vi "Update DelaysHW.vi"(8 "error in (no error)":errorcluster, 11 "BME_DG_System in":refnum<class "BME_DG_System.lvclass">) -> (0 "error out":errorcluster, 3 "BME_DG_System out":refnum<class "BME_DG_System.lvclass">)   [LabVIEW 2009, in "POLARIS BME DG.lvlib" / "BME_DG_System.lvclass"]
uses:
  BME_DG_System.lvclass
  BME_DG_System.lvclass/BME_DG_System.ctl
  BME_DG_Base/BME_DG_Base.lvclass
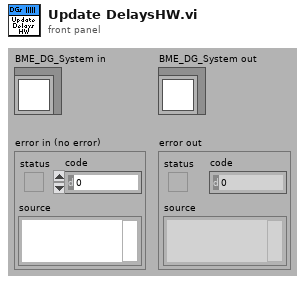
[diagram p1: front panel]
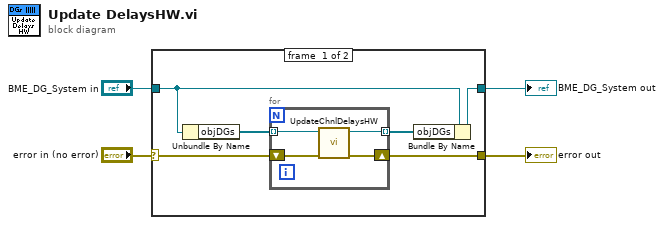
[diagram p0: block diagram]
diagram:
  n1 = case shown="No Error" "error in (no error)" {
    selector: "error in (no error)" -> [w8 w16]
    tunnel: [w5 w16] -> w3
    tunnel: [w7 w15] -> w1
    tunnel: "BME_DG_System in" -> [w10 w15]
    frame #0 {
      n2 = Unbundle By Name(w10) -> ("objDGs"=w9:refnum<class "BME_DG_Base.lvclass">[])
      n3 = for {
        tunnel: w9 -> [w14] mode=indexing
        tunnel: [w12] -> w6 mode=indexing
        shift-right: [w11] -> w5
        shift-left: w8 -> [w13]
        n4 = call "UpdateChnlDelaysHW.vi"("error in (no error)"=w13, "BME_DG_Base in"=w14) -> ("error out"=w11:errorcluster, "BME_DG_Base out"=w12:refnum<class "BME_DG_Base.lvclass">)  [unwired: 8 in]
      }
      n5 = Bundle By Name(cluster=w10, "objDGs"=w6) -> (w7:refnum<class "BME_DG_System.lvclass">)
    }
    frame #1 {
    }
  }
  "error out" <- w3
  "BME_DG_System out" <- w1
